vi "Write 1D History Point Arrary to NT Table.vi"   [LabVIEW 2016]
uses:
  <vilib>/Rock Robotics/Network Tables/NT Write Numeric Array.vi
types:
  T1 = cluster{"Yaw":dbl, "Roll":dbl, "Pitch":dbl, "Heading":dbl, "Fused Heading":dbl}
  T2 = cluster{"Quat W":dbl, "Quat X":dbl, "Quat Y":dbl, "Quat Z":dbl}
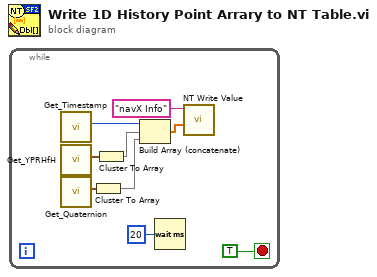
[diagram p0: block diagram]
diagram:
  n1 = while {
    stop <- TRUE stop-if-true
    n2 = call "Get_Timestamp.vi"() -> ("Timestamp"=w4:u32)  [unwired: 11 in]
    n3 = call "Get_YPRHfH.vi"() -> ("YRPHfH"=w7:T1)  [unwired: 11 in]
    n4 = call "Get_Quaternion.vi"() -> ("Quaternion"=w8:T2)  [unwired: 11 in]
    n5 = Cluster To Array(cluster=w8) -> (array=w5:dbl[])
    n6 = Cluster To Array(cluster=w7) -> (array=w6:dbl[])
    n7 = Build Array (concatenate)(w4, w6, w5) -> (w3:dbl[])
    n8 = Wait (ms)(milliseconds to wait=u32 20) -> ()  [unwired: 1 out]
    n9 = call-poly <vilib>:"NT Write Value.vi"("Numeric Array"=w3, "Name"="navX Info") -> ()  [unwired: 9 in, 1 out]
  }
